vi "Relay Out.vi"(2 "Relay Amp (%)":dbl format="%.2f", 3 "noise disturbance %":dbl format="%.2f", 4 "setpoint %":dbl=20.0 format="%.2f", 5 "PV %":dbl=20.0 format="%.2f") -> (0 "Zero Crossing":bool, 1 "relay output":dbl=50.0 format="%.2f")   [LabVIEW 2017, in "NI_PID__autopid compat.lvlib"]
doc: "This function relays the setpoint between (setpoint - relay amplitude) and (setpoint + relay amplitude)."
uses:
  <vilib>/addons/control/pid/NI_PID__autopid compat.lvlib
panel:
  # "Relay Out"
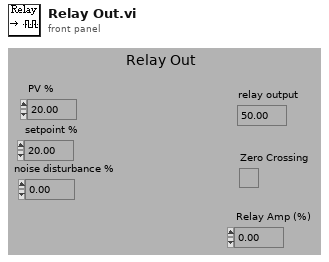
[diagram p1: front panel]
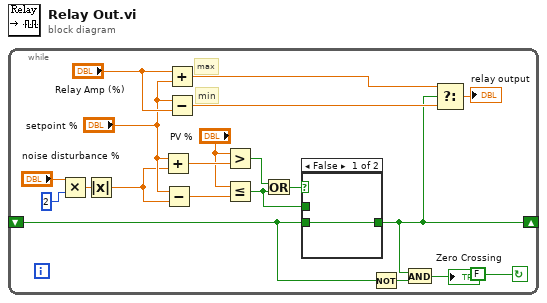
[diagram p0: block diagram]
diagram:
  n1 = while {
    shift-left: _ -> [w3]
    shift-right: [w2] -> _
    stop <- FALSE continue-if-true
    # "min"
    # "max"
    n2 = Multiply(x="noise disturbance %", y=2) -> (x*y=w17:dbl)
    n3 = Absolute Value(x=w17) -> (abs(x)=w12:dbl)
    n4 = Add(x="setpoint %", y=w12) -> (x+y=w20:dbl)
    n5 = Subtract(x="setpoint %", y=w12) -> (x-y=w11:dbl)
    n6 = Add(x="Relay Amp (%)", y="setpoint %") -> (x+y=w7:dbl)
    n7 = Subtract(x="setpoint %", y="Relay Amp (%)") -> (x-y=w6:dbl)
    n8 = Greater?(x="PV %", y=w20) -> (0:w9:bool)
    n9 = Less Or Equal?(x="PV %", y=w11) -> (x <= y?=w4:bool)
    n10 = Or(x=w9, y=w4) -> (x .or. y?=w5:bool)
    n11 = case shown="False" w5 {
      tunnel: w3 -> [w21 _]
      tunnel: [w21 w22] -> w2
      tunnel: w4 -> [_ w22]
      frame False {
      }
      frame True {
      }
    }
    n12 = Not(x=w3) -> (.not. x?=w18:bool)
    n13 = And(x=w2, y=w18) -> (x .and. y?=→"Zero Crossing":bool)
    n14 = Select(t=w7, s=w2, f=w6) -> (s? t:f=→"relay output":dbl)
  }
